vi "Regedit.vi"() -> ()   [LabVIEW 2020]
uses:
  <vilib>/registry/registry.llb/Registry SAM.ctl
  <vilib>/registry/registry.llb/Registry RtKey.ctl
  <vilib>/registry/registry.llb/Write Registry Value Simple STR.vi
  <vilib>/registry/registry.llb/Read Registry Value Simple STR.vi
panel:
  out "String/Binary data 2":string
  out "String/Binary data":string[](array[string])
  out "DWORD data":u32[](array[numeric])
  out "simple data types":enum16{"String", "Binary", "DWORD"}[](array[ring])
  out "class":string
  out "value info":T1
  out "values":string[](array[string])
  out "error out":errorcluster
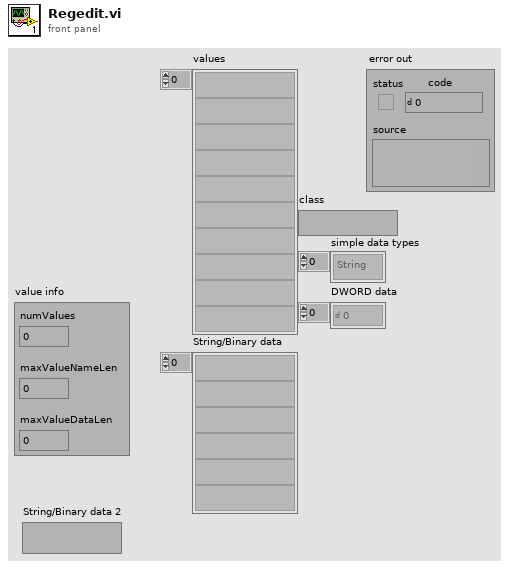
[diagram p1: front panel]
types:
  T1 = cluster{"numValues":i32, "maxValueNameLen":i32, "maxValueDataLen":i32}
  T2 = typedef "Registry RtKey.ctl" = enum32{"HKEY_CLASSES_ROOT", "HKEY_CURRENT_USER", "HKEY_LOCAL_MACHINE", "HKEY_USERS", "HKEY_PERFORMANCE_DATA", "HKEY_CURRENT_CONFIG", "HKEY_DYN_DATA"}
  T3 = typedef "Registry SAM.ctl" = enum32{"KEY_QUERY_VALUE", "KEY_SET_VALUE", "KEY_CREATE_SUB_KEY", "KEY_ENUMERATE_SUB_KEYS", "KEY_NOTIFY", "KEY_CREATE_LINK", "KEY_READ", "KEY_WRITE", "KEY_ALL_ACCESS", "KEY_READ | KEY_WRITE"}
  T4 = typedef "Registry refnum.ctl" = refnum<k1>
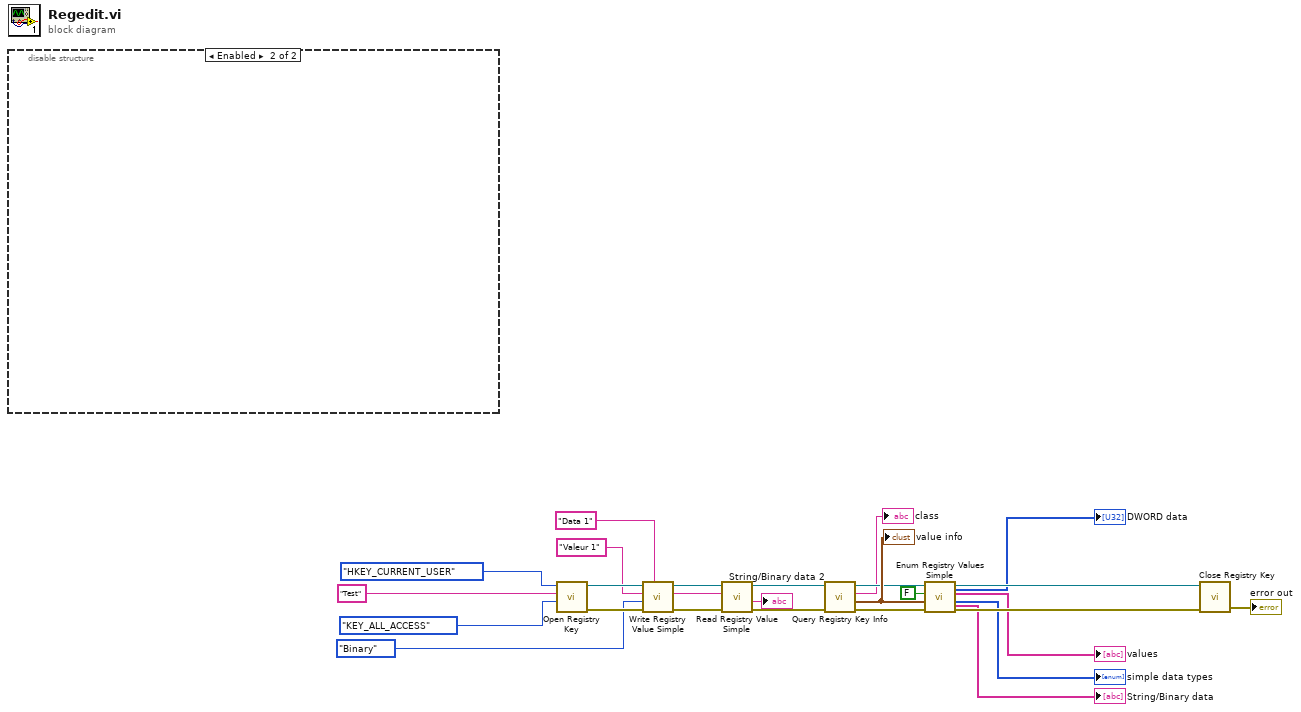
[diagram p0: block diagram]
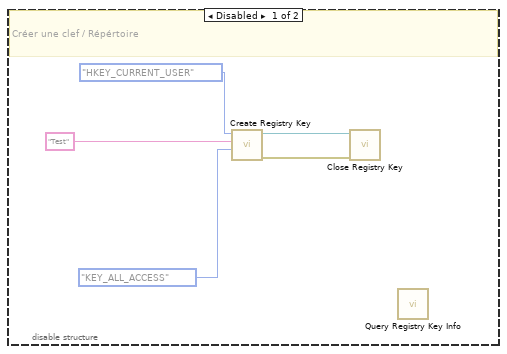
[diagram p2: hidden frame]
diagram:
  w5 = "Valeur 1" ("value")
  n1 = disable-structure shown="Enabled" {
    frame Disabled {
      # "Créer une clef / Répértoire"
      n2 = call <vilib>:"Create Registry Key.vi"("security access mask (KEY_READ | KEY_WRITE)"=Registry_SAM."KEY_ALL_ACCESS", "subkey"="Test", "root key (HKEY_LOCAL_MACHINE)"=Registry_RtKey."HKEY_CURRENT_USER") -> ("error out"=w27:errorcluster, "refnum out"=w26:T4)  [unwired: 6 in, 1 out]
      n3 = call <vilib>:"Close Registry Key.vi"("error in (no error)"=w27, "refnum"=w26) -> ()  [unwired: 5 in, 1 out]
      n4 = call <vilib>:"Query Registry Key Info.vi"() -> ()  [unwired: 7 in, 5 out]
    }
    frame Enabled {
    }
  }
  n5 = call <vilib>:"Open Registry Key.vi"("security access mask (KEY_READ | KEY_WRITE)"=Registry_SAM."KEY_ALL_ACCESS", "subkey"="Test", "root key (HKEY_LOCAL_MACHINE)"=Registry_RtKey."HKEY_CURRENT_USER") -> ("error out"=w20:errorcluster, "refnum out"=w21:T4)  [unwired: 7 in]
  n6 = call-poly <vilib>:"Write Registry Value Simple.vi"("String/Binary data"="Data 1", "error in (no error)"=w20, "simple data type"=enum16{"String", "Binary", "DWORD"}."Binary", "value"=w5, "refnum"=w21) -> ("error out"=w3:errorcluster, "refnum out"=w6:T4)  [unwired: 3 in]
  n7 = call-poly <vilib>:"Read Registry Value Simple.vi"("error in (no error)"=w3, "value"=w5, "refnum"=w6) -> ("error out"=w2:errorcluster, "String/Binary data"=→"String/Binary data 2":string, "refnum out"=w1:T4)  [unwired: 3 in, 1 out]
  n8 = call <vilib>:"Query Registry Key Info.vi"("error in (no error)"=w2, "refnum"=w1) -> ("error out"=w12:errorcluster, "value info"=w14:T1, "class"=→"class":string, "refnum out"=w13:T4)  [unwired: 5 in, 1 out]
  "value info" <- w14
  n9 = call <vilib>:"Enum Registry Values Simple.vi"("error in (no error)"=w12, "value info"=w14, "retrieve data? (F)"=FALSE, "refnum"=w13) -> ("error out"=w17:errorcluster, "simple data types"=→"simple data types":enum16{"String", "Binary", "DWORD"}[], "values"=→"values":string[], "refnum out"=w16:T4, "String/Binary data"=→"String/Binary data":string[], "DWORD data"=→"DWORD data":u32[])  [unwired: 2 in]
  n10 = call <vilib>:"Close Registry Key.vi"("error in (no error)"=w17, "refnum"=w16) -> ("error out"=→"error out":errorcluster)  [unwired: 5 in]
